vi "Tcp Daemon.vi"(11 "Http Port":u16) -> ()   [LabVIEW 2021, in "HttpServer.lvlib"]
uses:
  HttpServer.lvlib
  TypeDefs/Action.ctl
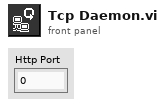
[diagram p1: front panel]
types:
  T1 = cluster{"Conn":refnum<k5>, "Last":timestamp, "Cnt":u32}
  T2 = typedef "HttpServer.lvlib/Action.ctl" = enum8{"noop", "add", "get", "set", "remove"}
  T3 = typedef "HttpServer.lvlib/WSGI.ctl" = cluster{"Header-Line":string, "Headers":map{string, string}, "Content":string}
  T4 = cluster{"Conn":refnum<k5>, "Last":timestamp, "Cnt":u32}[]
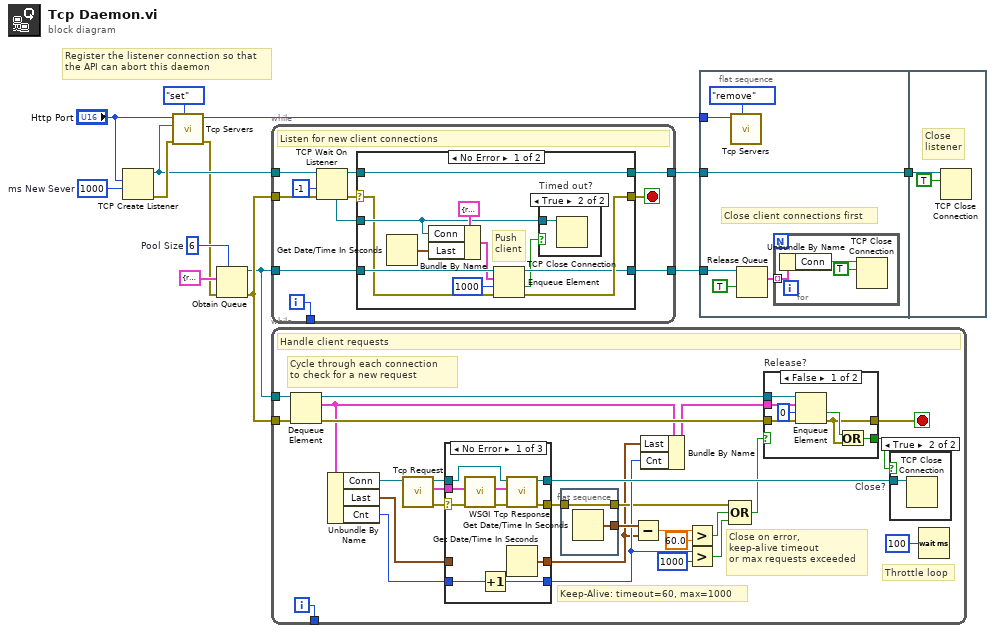
[diagram p0: block diagram]
diagram:
  w6 = 6  # Pool Size
  w13 = 1000  # ms New Sever
  # "Register the listener connection so that\nthe API can abort this daemon"
  n1 = TCP Create Listener(9:w13, 10:"Http Port") -> (0:w11:errorcluster, 3:w9:refnum<k5>)  [unwired: 3 in, 1 out]
  n2 = call "Tcp Servers.vi"("Action"=Action."set", "error in (no error)"=w11, "Connection in"=w9, "Server Port in"="Http Port") -> ("error out"=w5:errorcluster, "Server Port out"=w2:u16)  [unwired: 4 in, 2 out]
  n3 = Obtain Queue(max queue size (-1, unlimited)=w6, element data type=T1 {"Conn"=refnum, "Last"=timestamp(0 s since 1904-01-01), "Cnt"=0} ("Client"), error in (no error)=w5) -> (queue out=w3:refnum<queue>, error out=w4:errorcluster)  [unwired: 2 in, 1 out]
  n4 = while {
    tunnel: w9 -> [w25]
    tunnel: w4 -> [w18]
    tunnel: [w20] -> w14
    tunnel: w3 -> [w17]
    tunnel: [w16] -> w1
    tunnel: [w15] -> _
    i -> [w15]
    stop <- w22 stop-if-true
    # "Listen for new client connections"
    n5 = TCP Wait On Listener(8:w18, 9:-1 ("timeout ms (wait forever: -1)"), 11:w25) -> (0:w23:errorcluster, 3:w19:refnum<k5>, 4:w24:refnum<k5>)  [unwired: 1 in, 2 out]
    n6 = case shown="No Error" w23 {
      selector: w23 -> [w30 w40]
      tunnel: w24 -> [w32 _]
      tunnel: [w29 w40] -> w22
      tunnel: [w36 w39] -> w20
      tunnel: w19 -> [w36 w39]
      tunnel: w17 -> [w35 w38]
      tunnel: [w27 w38] -> w16
      frame No Error {
        # "Push\nclient"
        n7 = Get Date/Time In Seconds() -> (seconds since 1Jan1904=w28:timestamp)
        n8 = Bundle By Name(cluster=T1 {"Conn"=refnum, "Last"=timestamp(0 s since 1904-01-01), "Cnt"=0} ("Client"), "Conn"=w32, "Last"=w28) -> (w33:T1)
        n9 = Enqueue Element(queue=w35, element=w33, timeout in ms (-1)=1000, error in (no error)=w30) -> (queue out=w27:refnum<queue>, timed out?=w26:bool, error out=w29:errorcluster)
        n10 = case "Timed out?" shown="True" w26 {
          tunnel: w32 -> [_ w37]
          frame False {
          }
          frame True {
            n11 = TCP Close Connection(connection ID=w37) -> ()  [unwired: 2 in, 2 out]
          }
        }
      }
      frame Default {
      }
    }
  }
  n12 = while {
    tunnel: w4 -> [w42]
    tunnel: w3 -> [w41]
    tunnel: [w43] -> _
    i -> [w43]
    stop <- w66 stop-if-true
    # "Keep-Alive: timeout=60, max=1000"
    # "Throttle loop"
    # "Cycle through each connection\nto check for a new request"
    # "Close on error,\nkeep-alive timeout\nor max requests exceeded"
    # "Handle client requests"
    n13 = Dequeue Element(queue=w41, error in (no error)=w42) -> (queue out=w65:refnum<queue>, element=w60:T1, error out=w64:errorcluster)  [unwired: 1 in, 1 out]
    n14 = Unbundle By Name(w60) -> ("Conn"=w59:refnum<k5>, "Last"=w50:timestamp, "Cnt"=w49:u32)
    n15 = call "Tcp Request.vi"("Conn in"=w59) -> ("error out"=w63:errorcluster, "WSGI Request"=w62:T3, "Conn out"=w61:refnum<k5>)  [unwired: 8 in]
    n16 = case shown="No Error" w63 {
      selector: w63 -> [w74 w84 _]
      tunnel: [w80 w83 w87] -> w67
      tunnel: w62 -> [w72 _ _]
      tunnel: w61 -> [w79 w83 w87]
      tunnel: [w78 w84 _] -> w45
      tunnel: w50 -> [_ w82 w86]
      tunnel: [w77 w82 w86] -> w44
      tunnel: [w75 w81 w85] -> w47
      tunnel: w49 -> [w76 w81 w85]
      frame No Error {
        n17 = call "WSGI.vi"("error in (no error)"=w74, "WSGI Request"=w72) -> ("error out"=w73:errorcluster, "WSGI Response"=w71:T3)  [unwired: 8 in]
        n18 = Increment(x=w76) -> (x+1=w75:u32)
        n19 = call "Tcp Response.vi"("error in (no error)"=w73, "WSGI Response"=w71, "Conn in"=w79) -> ("error out"=w78:errorcluster, "Conn out"=w80:refnum<k5>)  [unwired: 7 in]
        n20 = Get Date/Time In Seconds() -> (seconds since 1Jan1904=w77:timestamp)
      }
      frame Default {
      }
      frame Error {
        # "Timed Out"
      }
    }
    n21 = flat-sequence {
      tunnel: [w70] -> w48
      tunnel: [w69] -> w46
      tunnel: w45 -> [w69]
      frame #0 {
        n22 = Get Date/Time In Seconds() -> (seconds since 1Jan1904=w70:timestamp)
      }
    }
    n23 = Subtract(x=w48, y=w44) -> (x-y=w52:dbl)
    n24 = Bundle By Name(cluster=w60, "Last"=w44, "Cnt"=w47) -> (w58:T1)
    n25 = Greater?(x=w52, y=60.0) -> (0:w56:bool)
    n26 = Greater?(x=w47, y=u32 1000) -> (0:w57:bool)
    n27 = Compound Arithmetic op=OR(w46, w56, w57) -> (w55:bool)
    n28 = case "Release?" shown="False" w55 {
      selector: w55 -> [_ w95]
      tunnel: [w89 w96] -> w66
      tunnel: w64 -> [w93 w96]
      tunnel: w65 -> [w94 _]
      tunnel: w58 -> [w92 _]
      tunnel: [w88 w95] -> w54
      frame False {
        n29 = Enqueue Element(queue=w94, element=w92, timeout in ms (-1)=0, error in (no error)=w93) -> (timed out?=w90:bool, error out=w89:errorcluster)  [unwired: 1 out]
        n30 = Or(x=w90, y=w89) -> (x .or. y?=w88:bool)
      }
      frame True {
      }
    }
    n31 = case "Close?" shown="True" w54 {
      tunnel: w67 -> [_ w97]
      frame False {
      }
      frame True {
        n32 = TCP Close Connection(connection ID=w97) -> ()  [unwired: 2 in, 2 out]
      }
    }
    n33 = Wait (ms)(milliseconds to wait=u32 100) -> ()  [unwired: 1 out]
  }
  n34 = flat-sequence {
    tunnel: w14 -> [w103]
    tunnel: [w103] -> w8
    tunnel: w2 -> [w101]
    tunnel: w1 -> [w100]
    tunnel: w8 -> [w108]
    frame #0 {
      # "Close client connections first"
      n35 = call "Tcp Servers.vi"("Action"=Action."remove", "Server Port in"=w101) -> ()  [unwired: 6 in, 4 out]
      n36 = Release Queue(queue=w100, force destroy? (F)=TRUE) -> (remaining elements=w98:T4)  [unwired: 1 in, 2 out]
      n37 = for {
        tunnel: w98 -> [w106] mode=indexing
        n38 = Unbundle By Name(w106) -> ("Conn"=w105:refnum<k5>)
        n39 = TCP Close Connection(connection ID=w105, abort (F)=TRUE) -> ()  [unwired: 1 in, 2 out]
      }
    }
    frame #1 {
      # "Close\nlistener"
      n40 = TCP Close Connection(connection ID=w108, abort (F)=TRUE) -> ()  [unwired: 1 in, 2 out]
    }
  }
